vi "MDAQ_READ_Status.vi"(8 "error in":errorcluster, 9 "Status_Cluster IN":T1 {"GATESTOP" format="%04x"; "GATESTRT" format="%04x"; "AMPLITUDE" format="%04x"; "M_CYCLES" format="%04x"; "N_CYCLES" format="%04x"; "STEP" format="%04x"; "BASE" format="%04x"; "CHAN" format="%04x"}, 11 "VISA resource name":refnum<visa-resource-name>) -> (0 "error out":errorcluster, 1 "output cluster":T1 {"GATESTOP" format="%04x"; "GATESTRT" format="%04x"; "AMPLITUDE" format="%04x"; "M_CYCLES" format="%04x"; "N_CYCLES" format="%04x"; "STEP" format="%04x"; "BASE" format="%04x"; "CHAN" format="%04x"}, 3 "VISA resource name out":refnum<visa-resource-name>)   [LabVIEW 2021]
uses:
  Status_Cluster.ctl
  dfacd9d0-e592-4c9f-9d6b-37ae124cbe0a.vi
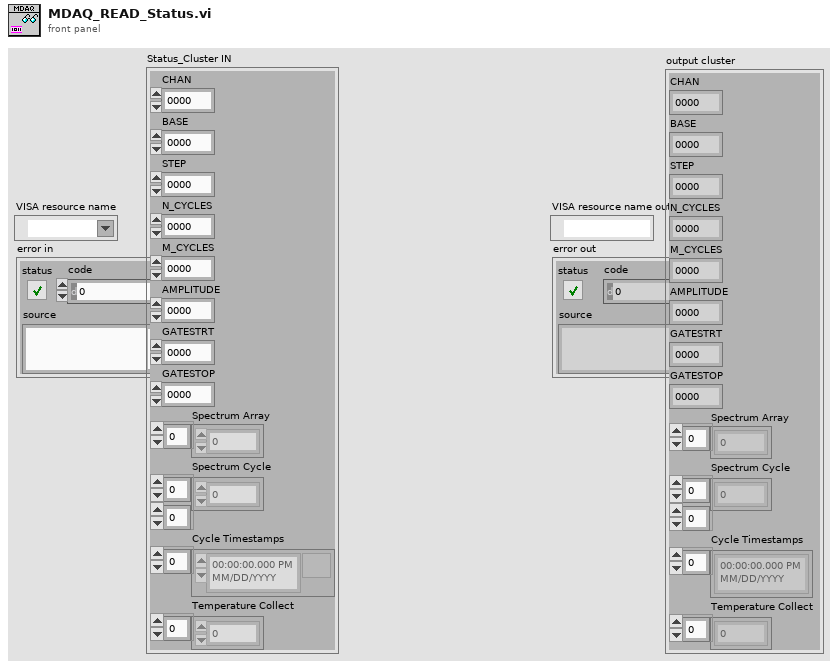
[diagram p1: front panel]
types:
  T1 = typedef "Status_Cluster.ctl" = cluster{"CHAN":u32, "BASE":u32, "STEP":u32, "N_CYCLES":u32, "M_CYCLES":u32, "AMPLITUDE":u32, "GATESTRT":u32, "GATESTOP":u32, "Spectrum Array":u32[], "Spectrum Cycle":u32[][], "Cycle Timestamps":timestamp[], "Temperature Collect":dbl[]}
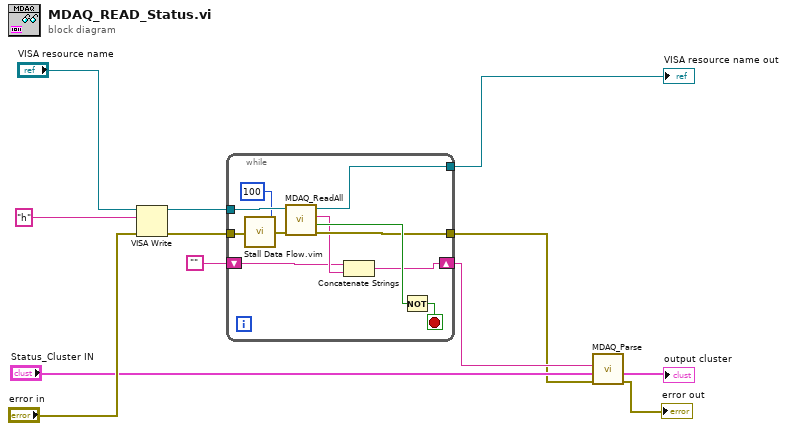
[diagram p0: block diagram]
diagram:
  n1 = VISA Write(VISA resource name="VISA resource name", write buffer="h", error in (no error)="error in") -> (VISA resource name out=w9:refnum<visa-resource-name>, error out=w1:errorcluster)  [unwired: 1 out]
  n2 = while {
    tunnel: w9 -> [w23]
    tunnel: [w22] -> w8
    tunnel: [w19] -> w4
    shift-right: [w16] -> w6
    shift-left: "" -> [w17]
    tunnel: w1 -> [w15]
    stop <- w21 stop-if-true
    n3 = call "Stall Data Flow.vim"("value in"=w15, "milliseconds to wait"=u32 100) -> ("value out"=w14:errorcluster)  [unwired: 1 out]
    n4 = call "MDAQ_ReadAll.vi"("error in"=w14, "VISA resource name"=w23) -> ("error IO"=w19:errorcluster, "Buffer Not Empty"=w20:bool, "read buffer"=w18:string, "VISA resource name out"=w22:refnum<visa-resource-name>)  [unwired: 6 in]
    n5 = Concatenate Strings(w17, w18) -> (w16:string)
    n6 = Not(x=w20) -> (.not. x?=w21:bool)
  }
  "VISA resource name out" <- w8
  n7 = call "MDAQ_Parse.vi"("error in"=w4, 9:"Status_Cluster IN", "input buffer"=w6) -> ("error out"=→"error out":errorcluster, "output cluster"=→"output cluster":T1)  [unwired: 7 in]
